vi "Move To.vi"(8 "error in (no error)":errorcluster, 10 "Hardware State":T1, 11 "New Position":dbl[](array[numeric])) -> (0 "error out":errorcluster, 2 "Hardware State Out":T1)   [LabVIEW 2015, in "XYZStage.lvlib"]
uses:
  XYZStage.lvlib
  XYZStage State.ctl
  XYZStage Loop State.ctl
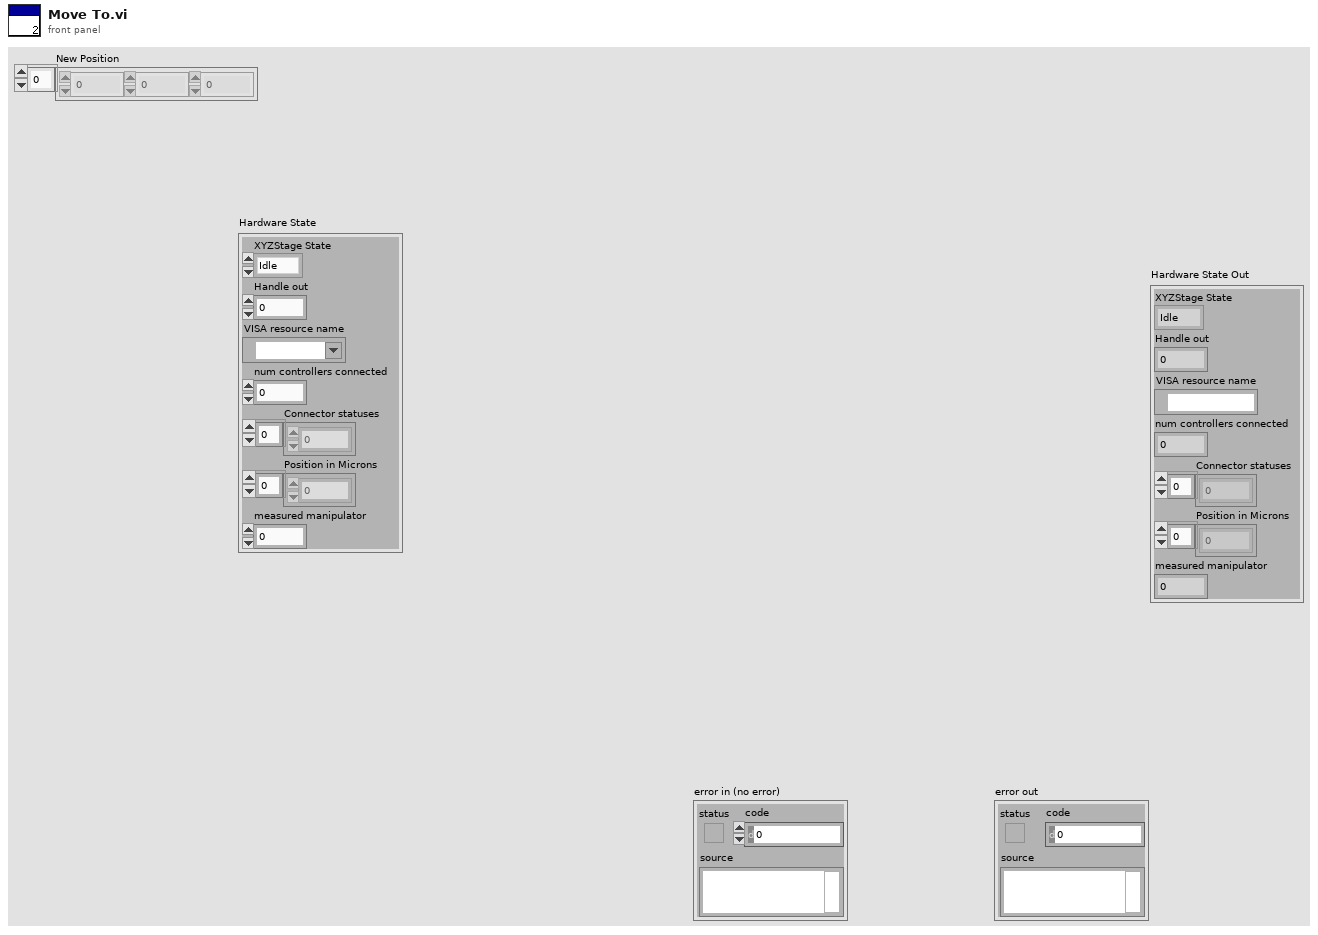
[diagram p1: front panel]
types:
  T1 = typedef "XYZStage.lvlib/XYZStage State.ctl" = cluster{"XYZStage State":T2, "Handle out":u32, "VISA resource name":refnum<visa-resource-name>, "num controllers connected":u8, "Connector statuses":u8[], "Position in Microns":dbl[], "measured manipulator":u8}
  T2 = typedef "XYZStage.lvlib/XYZStage Loop State.ctl" = enum16{"Idle", "Connected", "Moving"}
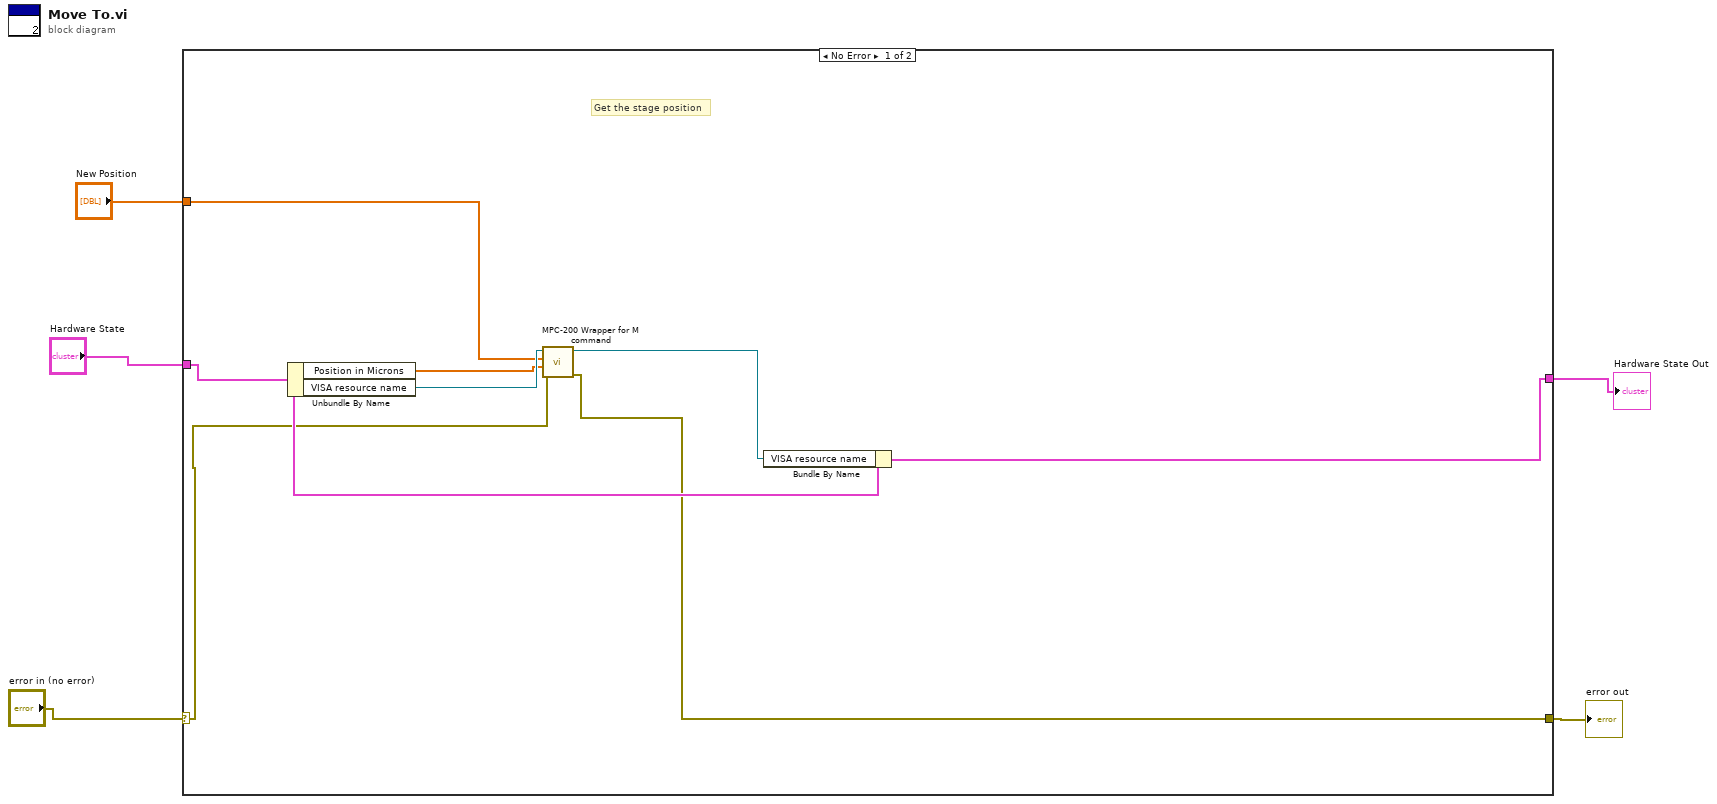
[diagram p0: block diagram]
diagram:
  n1 = case shown="No Error" "error in (no error)" {
    selector: "error in (no error)" -> [w8 w15]
    tunnel: [w9 w15] -> w4
    tunnel: [w12 w14] -> w3
    tunnel: "Hardware State" -> [w13 w14]
    tunnel: "New Position" -> [w7 _]
    frame No Error {
      # "Get the stage position"
      n2 = Unbundle By Name(w13) -> ("Position in Microns"=w6:dbl[], "VISA resource name"=w11:refnum<visa-resource-name>)
      n3 = call "MPC-200 Wrapper for M command.vi"("error in (no error)"=w8, "Current Position"=w6, "Move to Position"=w7, "VISA resource name in"=w11) -> ("error out"=w9:errorcluster, "VISA resource name out"=w10:refnum<visa-resource-name>)  [unwired: 6 in]
      n4 = Bundle By Name(cluster=w13, "VISA resource name"=w10) -> (w12:T1)
    }
    frame Error {
    }
  }
  "error out" <- w4
  "Hardware State Out" <- w3
